vi "Run Solver.vi"(7 "Debug Word (\"\")":string, 8 "error in":errorcluster, 10 "Number of Solves":i32=1, 11 "Solver":path) -> (0 "error out":errorcluster, 2 "Detailed Results":string, 3 "Average Number of Guesses":dbl)   [LabVIEW 2020, in "Wordle Engine.lvlib"]
uses:
  Wordle Engine.lvlib
panel:
  out "min # guesses":i32
  out "max # guesses":i32
  out "Current Solve":i32
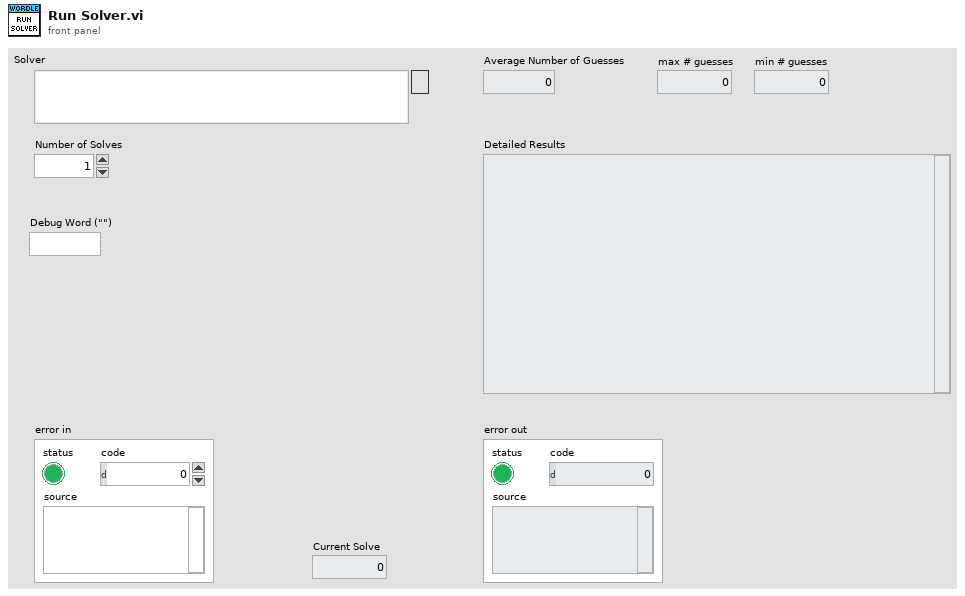
[diagram p1: front panel]
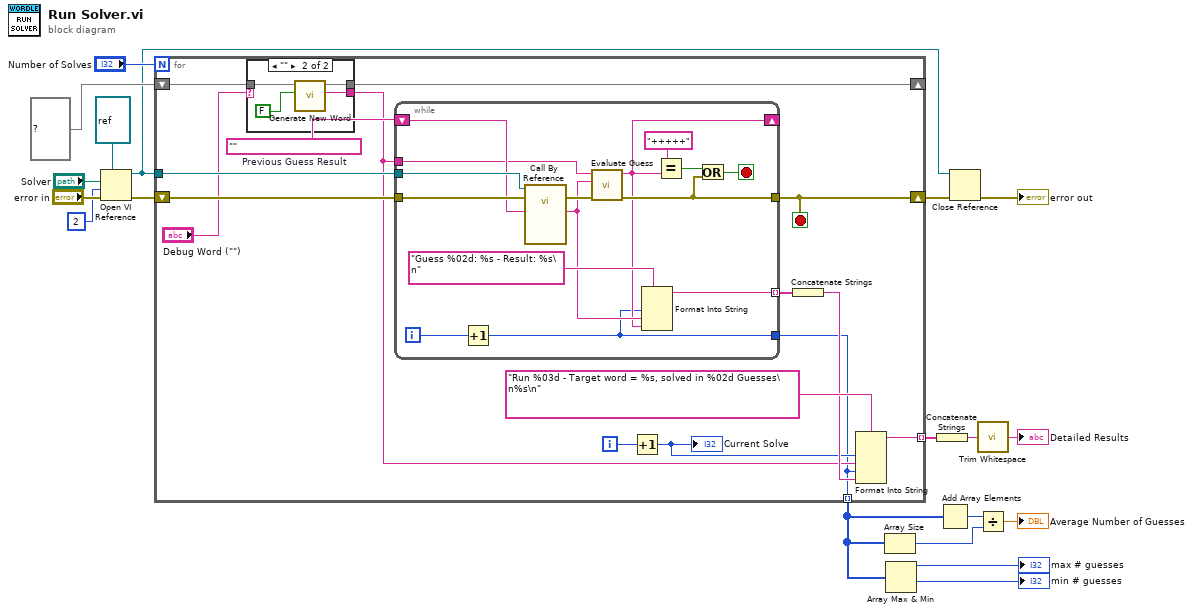
[diagram p0: block diagram]
diagram:
  n1 = Open VI Reference(type specifier VI Refnum (for type only)=refnum<vi> refnum, vi path="Solver", options=2, error in (no error)="error in") -> (vi reference=w7:refnum<vi>, error out=w16:errorcluster)  [unwired: 2 in]
  n2 = for {
    N: "Number of Solves" -> [_]
    tunnel: w7 -> [w34]
    shift-right: [w32] -> w14
    shift-left: w16 -> [w33]
    shift-right: [w29] -> _
    shift-left: set{string} {} ("Used Words in") -> [w30]
    tunnel: [w24] -> w10 mode=indexing
    tunnel: [w21] -> w3 mode=indexing
    i -> [w28]
    stop <- w32 stop-if-true
    w31 = ""  # Previous Guess Result
    n3 = case shown="\"\"" "Debug Word (\"\")" {
      selector: "Debug Word (\"\")" -> [w36 _]
      tunnel: w30 -> [w35 w40]
      tunnel: [w35 w38] -> w29
      tunnel: [w36 w37] -> w22
      frame Default {
      }
      frame "" {
        n4 = call "Generate New Word.vi"("Exclude Previously Selected Words"=FALSE, "Used Words in"=w40) -> ("Random Element"=w37:string, "Used Words out"=w38:set{string})  [unwired: 8 in]
      }
    }
    n5 = while {
      tunnel: w34 -> [w55]
      tunnel: w33 -> [w54]
      tunnel: [w49] -> w32
      shift-right: [w44] -> _
      shift-left: w31 -> [w53]
      tunnel: w22 -> [w52]
      tunnel: [w43] -> w26 mode=indexing
      tunnel: [w41] -> w21
      i -> [w42]
      stop <- w50 stop-if-true
      n6 = Increment(x=w42) -> (x+1=w41:i32)
      n7 = call-by-ref "?"(reference=w55, error in=w54, "Previous Guess Result"=w53) -> (error out=w51:errorcluster, "New Guess"=w45:string)  [unwired: 10 in, 1 out]
      n8 = call "Evaluate Guess.vi"("error in"=w51, "Guess"=w45, "Current Word"=w52) -> ("error out"=w49:errorcluster, "Result"=w44:string)  [unwired: 7 in]
      n9 = Format Into String(format string="Guess %02d: %s - Result: %s\n", w41, w45, w44) -> (resulting string=w43:string)  [unwired: 2 in, 1 out]
      n10 = Equal?(x="+++++", y=w44) -> (x = y?=w47:bool)
      n11 = Or(x=w47, y=w49) -> (x .or. y?=w50:bool)
    }
    n12 = Increment(x=w28) -> (x+1=w23:i32)
    "Current Solve" <- w23
    n13 = Concatenate Strings(w26) -> (w25:string)
    n14 = Format Into String(format string="Run %03d - Target word = %s, solved in %02d Guesses\n%s\n", w23, w22, w21, w25) -> (resulting string=w24:string)  [unwired: 2 in, 1 out]
  }
  n15 = Array Size(array=w3) -> (size(s)=w5:i32)
  n16 = Array Max & Min(array=w3) -> (max value=→"max # guesses":i32, min value=→"min # guesses":i32)  [unwired: 2 out]
  n17 = Concatenate Strings(w10) -> (w9:string)
  n18 = Add Array Elements(numeric array=w3) -> (sum=w6:i32)
  n19 = Close Reference(reference=w7, error in (no error)=w14) -> (error out=→"error out":errorcluster)
  n20 = call <vilib>:"Trim Whitespace.vi"("string"=w9) -> ("trimmed string"=→"Detailed Results":string)  [unwired: 1 in]
  n21 = Divide(x=w6, y=w5) -> (x/y=→"Average Number of Guesses":dbl)
